vi "MainPage Settings.vi"(7 "Action":T1, 8 "error in (no error)":errorcluster, 10 "Settings In":T3, 11 "Item Ref in":T2 format="%.0x") -> (0 "error out":errorcluster, 2 "Settings Out":T3, 3 "Item Ref out":T2 format="%.0x")   [LabVIEW 2026, in "WebPage Addon System Explorer.lvlib"]
uses:
  WebPage Addon System Explorer.lvlib
  Types/Main.Settings.ctl
  <vilib>/NI VeriStand/Custom Device API/Custom Device Item Ref.ctl
  Types/Page Settings Action.ctl
  Addon Shared/Constants.vi
  <vilib>/NI VeriStand/Custom Device API/Get Item Property (Double).vi
  <vilib>/NI VeriStand/Custom Device API/Get Item Property (U32).vi
  <vilib>/NI VeriStand/Custom Device API/Get Item Property (String).vi
  <vilib>/NI VeriStand/Custom Device API/Set Item Property (Double).vi
  <vilib>/NI VeriStand/Custom Device API/Set Item Property (U32).vi
  <vilib>/NI VeriStand/Custom Device API/Set Item Property (String).vi
  <vilib>/NI VeriStand/Custom Device API/Custom Device API.lvlib
  Addon Shared/WebPage Addon Shared.lvlib
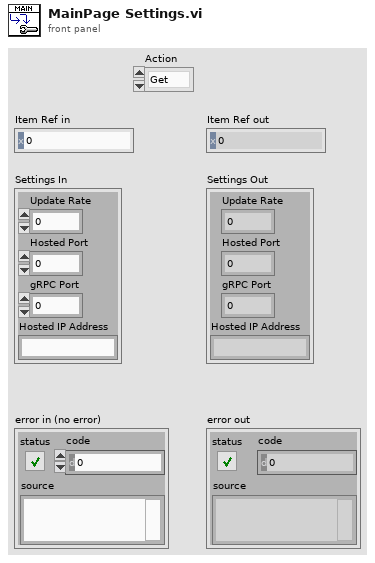
[diagram p1: front panel]
types:
  T1 = typedef "WebPage Addon System Explorer.lvlib/Page Settings Action.ctl" = enum16{"Get", "Set"}
  T2 = typedef "Custom Device API.lvlib/Custom Device Item Ref.ctl" = u64
  T3 = typedef "WebPage Addon System Explorer.lvlib/Main.Settings.ctl" = cluster{"Update Rate":dbl, "Hosted Port":u32, "gRPC Port":u32, "Hosted IP Address":string}
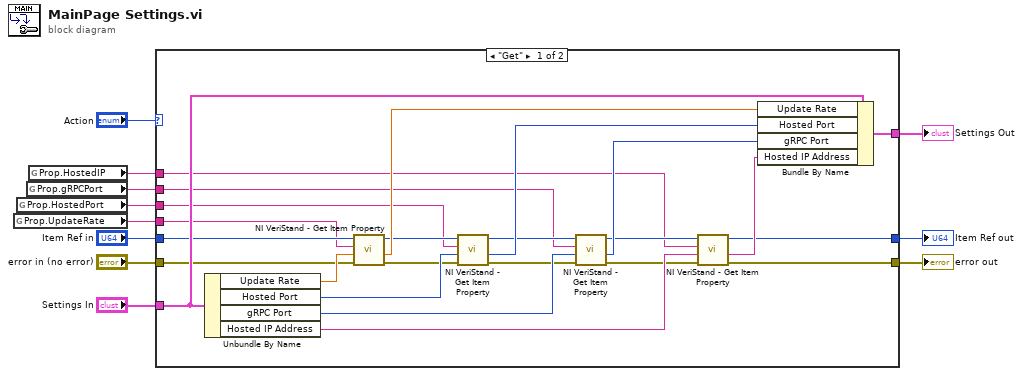
[diagram p0: block diagram]
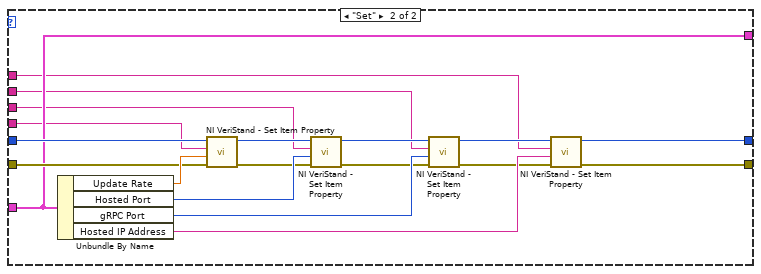
[diagram p2: hidden frame]
diagram:
  n1 = global read "Constants.vi" "Prop.UpdateRate"() -> (w2:string)
  n2 = global read "Constants.vi" "Prop.HostedPort"() -> (w5:string)
  n3 = global read "Constants.vi" "Prop.gRPCPort"() -> (w4:string)
  n4 = global read "Constants.vi" "Prop.HostedIP"() -> (w3:string)
  n5 = case shown="\"Get\"" "Action" {
    tunnel: [w35 w40] -> w11
    tunnel: "Settings In" -> [w30 w40]
    tunnel: [w25 w50] -> w9
    tunnel: [w24 w49] -> w8
    tunnel: "Item Ref in" -> [w17 w42]
    tunnel: "error in (no error)" -> [w16 w41]
    tunnel: w5 -> [w14 w39]
    tunnel: w4 -> [w13 w38]
    tunnel: w3 -> [w12 w37]
    tunnel: w2 -> [w15 w36]
    frame "Get" {
      n6 = Unbundle By Name(w30) -> ("Update Rate"=w26:dbl, "Hosted Port"=w27:u32, "gRPC Port"=w28:u32, "Hosted IP Address"=w29:string)
      n7 = call-poly <vilib>:"NI VeriStand - Get Item Property.vi"("error in (no error)"=w16, "Default Value"=w26, "Property Name"=w15, "Item Ref in"=w17) -> ("error out"=w18:errorcluster, "Value"=w31:dbl, "Item Ref out"=w19:T2)  [unwired: 4 in, 1 out]
      n8 = call-poly <vilib>:"NI VeriStand - Get Item Property.vi"("error in (no error)"=w18, "Default Value"=w27, "Property Name"=w14, "Item Ref in"=w19) -> ("error out"=w22:errorcluster, "Value"=w32:u32, "Item Ref out"=w20:T2)  [unwired: 4 in, 1 out]
      n9 = call-poly <vilib>:"NI VeriStand - Get Item Property.vi"("error in (no error)"=w22, "Default Value"=w28, "Property Name"=w13, "Item Ref in"=w20) -> ("error out"=w23:errorcluster, "Value"=w33:u32, "Item Ref out"=w21:T2)  [unwired: 4 in, 1 out]
      n10 = call-poly <vilib>:"NI VeriStand - Get Item Property.vi"("error in (no error)"=w23, "Default Value"=w29, "Property Name"=w12, "Item Ref in"=w21) -> ("error out"=w24:errorcluster, "Value"=w34:string, "Item Ref out"=w25:T2)  [unwired: 4 in, 1 out]
      n11 = Bundle By Name(cluster=w30, "Update Rate"=w31, "Hosted Port"=w32, "gRPC Port"=w33, "Hosted IP Address"=w34) -> (w35:T3)
    }
    frame "Set" {
      n12 = Unbundle By Name(w40) -> ("Update Rate"=w51:dbl, "Hosted Port"=w52:u32, "gRPC Port"=w53:u32, "Hosted IP Address"=w54:string)
      n13 = call-poly <vilib>:"NI VeriStand - Set Item Property.vi"("error in (no error)"=w41, "Value"=w51, "Property Name"=w36, "Item Ref in"=w42) -> ("error out"=w43:errorcluster, "Item Ref out"=w44:T2)  [unwired: 5 in, 1 out]
      n14 = call-poly <vilib>:"NI VeriStand - Set Item Property.vi"("error in (no error)"=w43, "Value"=w52, "Property Name"=w39, "Item Ref in"=w44) -> ("error out"=w47:errorcluster, "Item Ref out"=w45:T2)  [unwired: 5 in, 1 out]
      n15 = call-poly <vilib>:"NI VeriStand - Set Item Property.vi"("error in (no error)"=w47, "Value"=w53, "Property Name"=w38, "Item Ref in"=w45) -> ("error out"=w48:errorcluster, "Item Ref out"=w46:T2)  [unwired: 5 in, 1 out]
      n16 = call-poly <vilib>:"NI VeriStand - Set Item Property.vi"("error in (no error)"=w48, "Value"=w54, "Property Name"=w37, "Item Ref in"=w46) -> ("error out"=w49:errorcluster, "Item Ref out"=w50:T2)  [unwired: 5 in, 1 out]
    }
  }
  "Settings Out" <- w11
  "Item Ref out" <- w9
  "error out" <- w8
